vi "RPM to RadsPerSecond.vi"(11 "Desired RPM":dbl) -> (3 "Numeric":dbl)   [LabVIEW 2015]
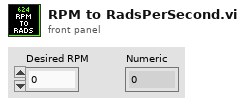
[diagram p1: front panel]
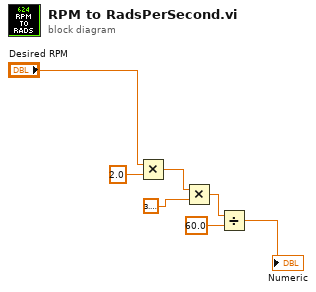
[diagram p0: block diagram]
diagram:
  n1 = Multiply(x="Desired RPM", y=2.0) -> (x*y=w2:dbl)
  n2 = Multiply(x=w2, y=3.141592653589793) -> (x*y=w4:dbl)
  n3 = Divide(x=w4, y=60.0) -> (x/y=→"Numeric":dbl)
